vi "One Dir Up.vi"(11 "Current dir":string) -> (2 "Top Directory?":bool, 3 "One up dir":string)   [LabVIEW 2021]
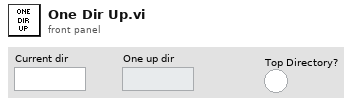
[diagram p1: front panel]
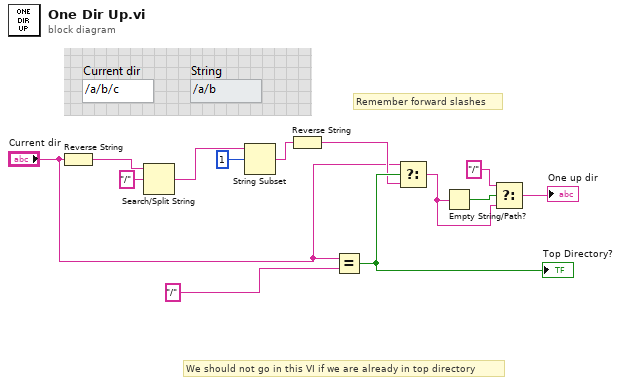
[diagram p0: block diagram]
diagram:
  # "We should not go in this VI if we are already in top directory"
  # "Remember forward slashes"
  n1 = Reverse String(1:"Current dir") -> (0:w10:string)
  n2 = Search/Split String(string=w10, search string/char (-)="/") -> (match + rest of string=w6:string)  [unwired: 1 in, 2 out]
  n3 = String Subset(string=w6, offset (0)=1) -> (substring=w13:string)  [unwired: 1 in]
  n4 = Reverse String(1:w13) -> (0:w7:string)
  n5 = Equal?(x="Current dir", y="/") -> (x = y?=w8:bool)
  "Top Directory?" <- w8
  n6 = Select(t="Current dir", s=w8, f=w7) -> (s? t:f=w1:string)
  n7 = Empty String/Path?(string/path=w1) -> (empty?=w4:bool)
  n8 = Select(t="/", s=w4, f=w1) -> (s? t:f=→"One up dir":string)
